vi "Clear All Discretes.vi"(8 "error in":errorcluster, 11 "DIG_IO in":refnum<class "DIG_IO.lvclass">) -> (0 "error out":errorcluster, 3 "DIG_IO out":refnum<class "DIG_IO.lvclass">)   [LabVIEW 2019, in "DIG_IO.lvlib" / "DIG_IO.lvclass"]
uses:
  Library/DIG_IO.lvclass
  C:/Users/Public/Documents/Development/builds/Engine/Monitored Actor.lvlibp/Monitored Actor/Monitored Actor/Monitored Actor.lvclass
  C:/Users/Public/Documents/Development/builds/Instruments/Instruments.lvlibp/Library/Instruments.lvclass
  Library/DIG_IO.lvclass/DIG_IO.ctl
  Accessors/Read Digital.vi
  Accessors/Write Digital.vi
  builds/Engine/Monitored Actor.lvlibp/Monitored Actor/Monitored Actor/Read Actor Label.vi
  builds/Instruments/Instruments.lvlibp/Private/Polymorphic/Special/Event from String.vi
  builds/Instruments/Instruments.lvlibp/Accessors/Command with Logging.vi
  builds/Instruments/Instruments.lvlibp/Library/Instruments.lvclass
  builds/Instruments/Instruments.lvlibp
  builds/Engine/Engine.lvlibp/Project/Engine.lvclass
  C:/Users/Public/Documents/Development/builds/Engine/Engine.lvlibp/Project/Engine.lvclass
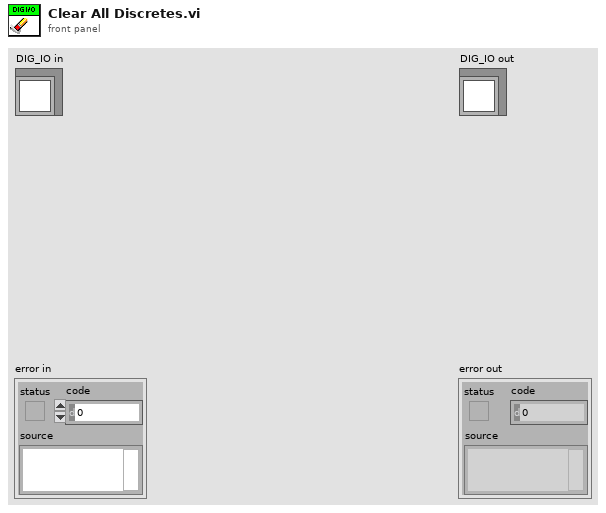
[diagram p1: front panel]
types:
  T1 = cluster{"Timestamp":timestamp, "Description":string, "Data":string}
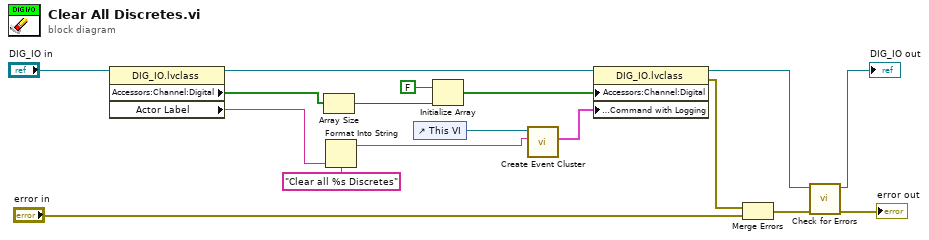
[diagram p0: block diagram]
diagram:
  n1 = property class="DIG_IO.lvclass"(reference="DIG_IO in") -> (reference out=w16:refnum<class "DIG_IO.lvclass">, "Accessors:Channel:Digital"=w14:bool[], "Actor Label"=w13:string)  [unwired: 1 in, 1 out]
  n2 = Array Size(array=w14) -> (size(s)=w11:i32)
  n3 = Format Into String(format string="Clear all %s Discretes", w13) -> (resulting string=w6:string)  [unwired: 2 in, 1 out]
  n4 = control-ref of="This VI"() -> (w12:refnum<vi>)
  n5 = Initialize Array(FALSE, w11) -> (w10:bool[])
  n6 = call-poly "Create Event Cluster.vi"("Value"=w6, "VI Refnum"=w12) -> ("Event Data"=w8:T1)  [unwired: 9 in]
  n7 = property class="DIG_IO.lvclass"(reference=w16, "Accessors:Channel:Digital"=w10, "Accessors:Logging:Command with Logging"=w8) -> (reference out=w2:refnum<class "DIG_IO.lvclass">, error out=w15:errorcluster)  [unwired: 1 in]
  n8 = Merge Errors(w15, "error in") -> (w5:errorcluster)
  n9 = call "Check for Errors.vi"("error in"=w5, "Engine in"=w2) -> ("error out"=→"error out":errorcluster, "Engine out"=→"DIG_IO out":refnum<class "DIG_IO.lvclass">)  [unwired: 8 in]
